vi "dummy menu vi.vi"() -> ()   [LabVIEW 2013, in "Logger.lvlib"]
uses:
  Logger.lvlib
panel:
  in  "Boolean":bool
  # "Dummy Menu VI"
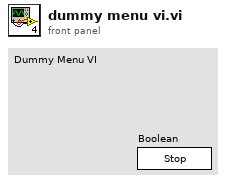
[diagram p1: front panel]
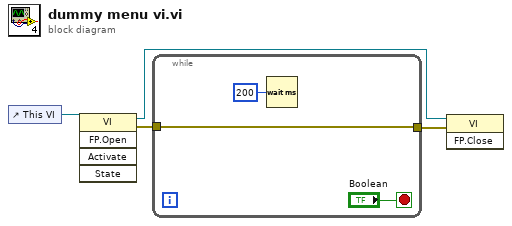
[diagram p0: block diagram]
diagram:
  n1 = control-ref of="This VI"() -> (w4:refnum<vi>)
  n2 = invoke class="VI" method="FP.Open"(reference=w4) -> (reference out=w2:refnum<vi>, error out=w3:errorcluster)  [unwired: 4 in, 3 out]
  n3 = while {
    tunnel: w3 -> [w5]
    tunnel: [w5] -> w1
    stop <- "Boolean" stop-if-true
    n4 = Wait (ms)(milliseconds to wait=u32 200) -> ()  [unwired: 1 out]
  }
  n5 = invoke class="VI" method="FP.Close"(reference=w2, error in=w1) -> ()  [unwired: 1 in, 3 out]
